vi "SetDrivePid.vi"(8 "error in (no error)":errorcluster, 9 "PID":T9, 10 "Profile Slot":u8 max=1, 11 "RobotDriveRef In":T1={"RobotDriveDevRef"={"DevStatus"={"status"=FALSE, "code"=0, "source"=""}, "Motors[]"=[], "Square Inputs"=FALSE, "Max Output"=1.0}, "Control Mode"=enum."Unchanged / Invalid"}) -> (0 "error out":errorcluster, 3 "RobotDriveRef Out":T1={"RobotDriveDevRef"={"DevStatus"={"status"=FALSE, "code"=0, "source"=""}, "Motors[]"=[], "Square Inputs"=FALSE, "Max Output"=1.0}, "Control Mode"=enum."Unchanged / Invalid"})   [LabVIEW 2015]
uses:
  PID Type Def.ctl
  RobotDrive Type Def.ctl
  <vilib>/Rock Robotics/WPI/MotorControl/WPI_MotorControlDeviceRef.ctl
  <vilib>/Rock Robotics/WPI/MotorControl/WPI_MotorControlType.ctl
  <vilib>/Rock Robotics/SystemInterfaces/DIO/FPGA_DIOPWMChannel.ctl
  <vilib>/Rock Robotics/WPI/PWM/WPI_PWMDeadband.ctl
  <vilib>/Rock Robotics/WPI/CAN/Jaguar/SubVIs/WPI_CANJaguar_ControlMode.ctl
  <vilib>/Rock Robotics/WPI/CAN/TalonSRX/WPI_CANTalonSRX_APIControlMode.ctl
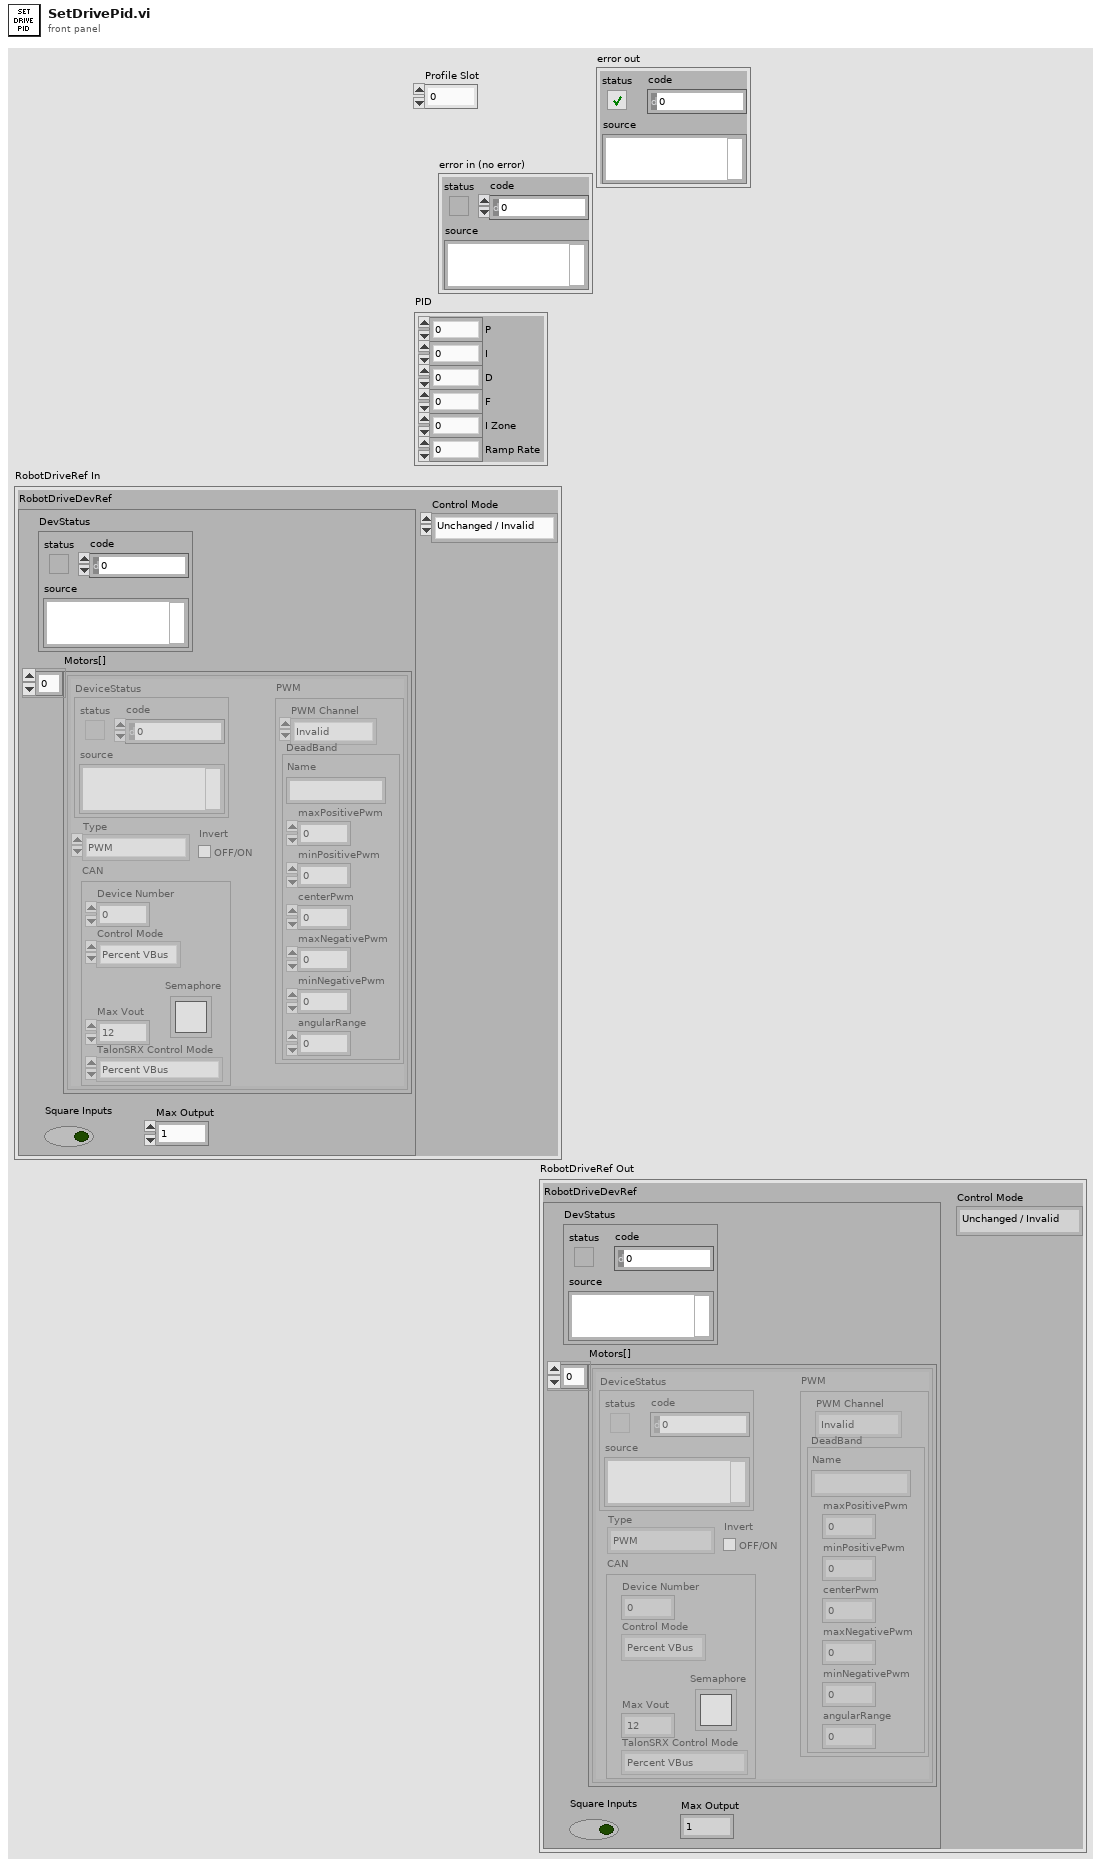
[diagram p1: front panel]
types:
  T1 = typedef "RobotDrive Type Def.ctl" = cluster{"RobotDriveDevRef":cluster{"DevStatus":errorcluster, "Motors[]":T2[], "Square Inputs":bool, "Max Output":dbl}, "Control Mode":T8}
  T2 = typedef "WPI_MotorControlDeviceRef.ctl" = cluster{"DeviceStatus":errorcluster, "Type":T3, "PWM":cluster{"PWM Channel":T4, "DeadBand":T5}, "CAN":cluster{"Device Number":u8, "Control Mode":T6, "Semaphore":T7, "Max Vout":dbl, "TalonSRX Control Mode":T8}, "Invert":bool}
  T3 = typedef "WPI_MotorControlType.ctl" = enum16{"PWM", "CAN", "CANTalonSRX"}
  T4 = typedef "FPGA_DIOPWMChannel.ctl" = enum8{"PWM 0", "PWM 1", "PWM 2", "PWM 3", "PWM 4", "PWM 5", "PWM 6", "PWM 7", "PWM 8", "PWM 9", "PWM MXP 0", "PWM MXP 1", "PWM MXP 2", "PWM MXP 3", "PWM MXP 4", "PWM MXP 5", "PWM MXP 6", "PWM MXP 7", "PWM MXP 8", "PWM MXP 9", "Invalid"}
  T5 = typedef "WPI_PWMDeadband.ctl" = cluster{"Name":string, "maxPositivePwm":i32, "minPositivePwm":i32, "centerPwm":i32, "maxNegativePwm":i32, "minNegativePwm":i32, "angularRange":u16}
  T6 = typedef "WPI_CANJaguar_ControlMode.ctl" = enum8{"Percent VBus", "Current", "Speed", "Position", "Voltage"}
  T7 = typedef "Semaphore RefNum" = refnum<k1>
  T8 = typedef "WPI_CANTalonSRX_APIControlMode.ctl" = enum8{"Percent VBus", "Speed", "Position", "Slave", "Unchanged / Invalid", "Voltage Compensation", "Current", "Motion Profile"}
  T9 = typedef "PID Type Def.ctl" = cluster{"P":dbl, "I":dbl, "D":dbl, "F":dbl, "I Zone":dbl, "Ramp Rate":dbl}
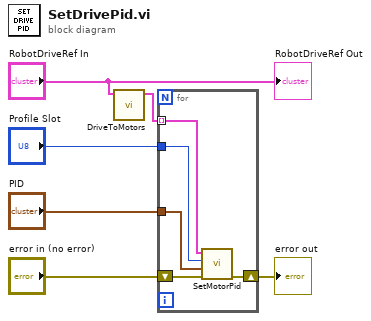
[diagram p0: block diagram]
diagram:
  n1 = call "DriveToMotors.vi"("RobotDriveRef"="RobotDriveRef In") -> ("Motors Out"=w6:T2[])  [unwired: 10 in]
  n2 = for {
    tunnel: w6 -> [w9] mode=indexing
    shift-right: [w10] -> w4
    shift-left: "error in (no error)" -> [w11]
    tunnel: "PID" -> [w8]
    tunnel: "Profile Slot" -> [w7]
    n3 = call "SetMotorPid.vi"("error in (no error)"=w11, "PID"=w8, "Parameter Slot"=w7, "Motor Ref In"=w9) -> ("error out"=w10:errorcluster)  [unwired: 6 in, 1 out]
  }
  "error out" <- w4
  "RobotDriveRef Out" <- "RobotDriveRef In"
